vi "rt_loop_data_acquisition_02_01.vi"(8 "error in (no error)":errorcluster caption="错误输入（无错误）", 11 "Message Queues":T1 caption="消息队列") -> (0 "error out":errorcluster caption="错误输出")   [LabVIEW 2015]
uses:
  support_vis/message_queue/all_rt_message_queues.ctl
  support_vis/message_queue/message_cluster.ctl
  globals/global_monitoring_variables.vi
  globals/global_configuration_options.vi
  support_vis/message_queue/message_queue.lvlib
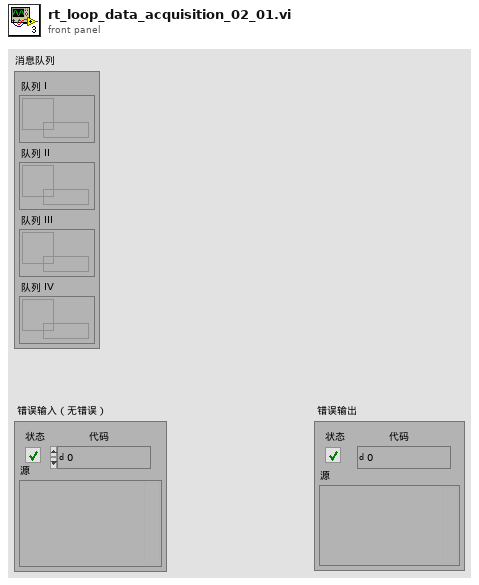
[diagram p1: front panel]
types:
  T1 = typedef "message_queue.lvlib/all_rt_message_queues.ctl" = cluster{"Queue I":refnum<queue>, "Queue II":refnum<queue>, "Queue III":refnum<queue>, "Queue IV":refnum<queue>}
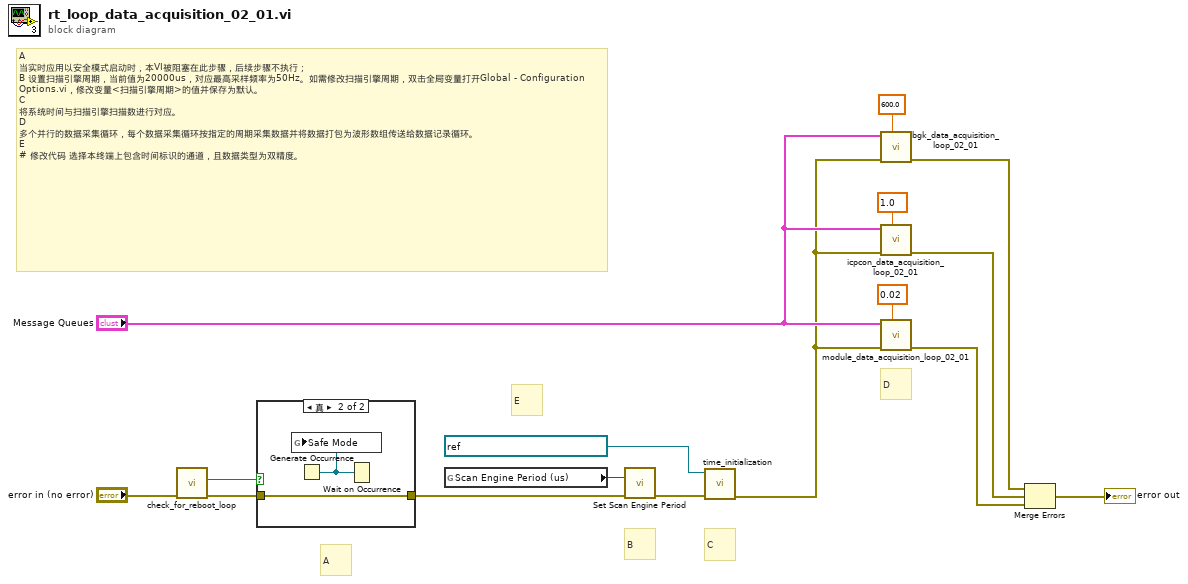
[diagram p0: block diagram]
diagram:
  # "E"
  # "D"
  # "C"
  # "B"
  # "A"
  # "A\n当实时应用以安全模式启动时，本VI被阻塞在此步骤，后续步骤不执行；\nB 设置扫描引擎周期，当前值为20000us，对应最高采样频率为50Hz。如需修改扫描引擎周期，双击全局变量打开Global - Configuration Options.vi，修改变量<扫描引擎周期>的值并保存为默认。\nC\n将系统时间与扫描引擎扫描数进行对应。\nD\n多个并行的数据采集循环，每个数据采集循环按指定的周期采集数据并将数据打包为波形数组传送给数据记录循环。\nE\n# 修改代码 选择本终端上包含时间标识的通道，且数据类型为双精度。"
  n1 = call "check_for_reboot_loop.vi"("error in (no error)"="error in (no error)") -> ("error out"=w13:errorcluster, "Start in Safe Mode?"=w14:bool)  [unwired: 9 in]
  n2 = case shown="真" w14 {
    tunnel: w13 -> [w17 w19]
    tunnel: [w17 w19] -> w7
    frame False {
    }
    frame True {
      n3 = Generate Occurrence() -> (w18:refnum<k4>)
      n4 = global write "global_monitoring_variables.vi" "Safe Mode"(w18) -> ()
      n5 = Wait on Occurrence(2:w18) -> ()  [unwired: 2 in, 1 out]
    }
  }
  n6 = global read "global_configuration_options.vi" "Scan Engine Period (us)"() -> (w5:u32)
  n7 = call <vilib>:"Set Scan Engine Period.vi"("scan period (uSec)"=w5, "error in (no error)"=w7) -> ("error out"=w6:errorcluster)  [unwired: 13 in]
  n8 = call "time_initialization.vi"("shared variable ref"=refnum<k21> "ni.var.io://ni-crio-9036-fcxf/Mod1/FCXF-X-02-A01", "error in (no error)"=w6) -> ("error out"=w8:errorcluster)  [unwired: 8 in]
  n9 = call "bgk_data_acquisition_loop_02_01.vi"("Period (s)"=600.0, "error in (no error)"=w8, "Message Queues"="Message Queues") -> ("error out"=w10:errorcluster)  [unwired: 8 in]
  n10 = call "icpcon_data_acquisition_loop_02_01.vi"("sampling period (s)"=1.0, "error in (no error)"=w8, "Message Queues"="Message Queues") -> ("error out"=w11:errorcluster)  [unwired: 8 in]
  n11 = call "module_data_acquisition_loop_02_01.vi"("Sampling Period (S)"=0.02 ("Sampling Period(S)"), "error in (no error)"=w8, "Message Queues"="Message Queues") -> ("error out"=w12:errorcluster)  [unwired: 8 in]
  n12 = Merge Errors(w10, w11, w12) -> (→"error out":errorcluster)
